vi "Virtual Index of Element in Incremental Array.vi"(9 "Value":dbl, 11 "Incremental Array":dbl[](array[numeric])) -> (0 "Valid Array":bool, 1 "Virtual Index":dbl)   [LabVIEW 2021, in "Arrays.lvlib"]
uses:
  Arrays.lvlib
  bfce6fbf-d7d3-4d45-9a31-a5a003d58b92.vi
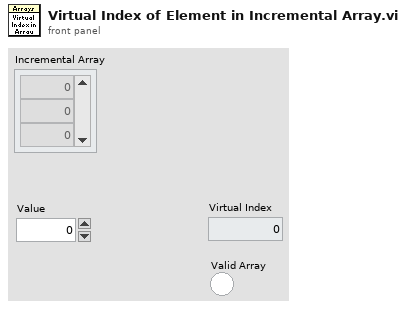
[diagram p1: front panel]
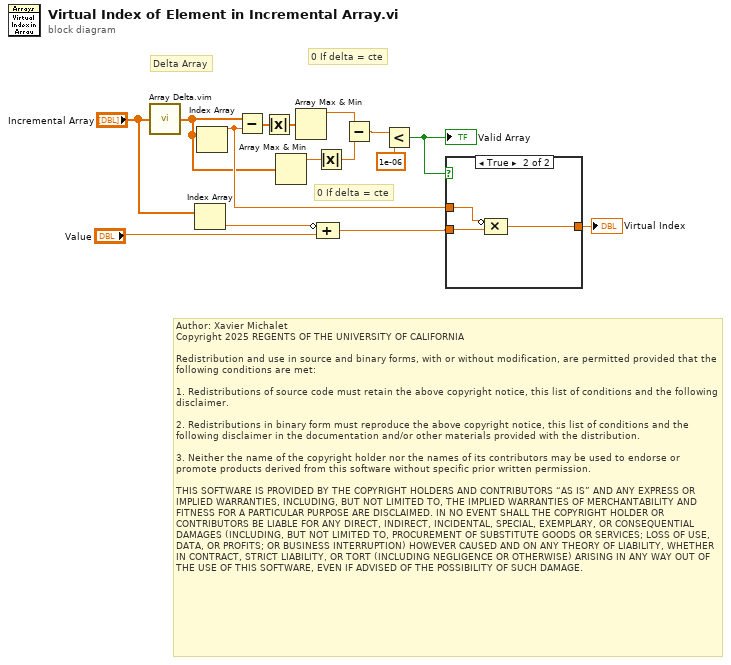
[diagram p0: block diagram]
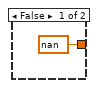
[diagram p2: hidden frame]
diagram:
  # "Author: Xavier Michalet\nCopyright 2025 REGENTS OF THE UNIVERSITY OF CALIFORNIA\n\nRedistribution and use in source and binary forms, with or without modification, are permitted provided that the following conditions are met:\n\n1. Redistributions of source code must retain the above copyright notice, this list of conditions and the following disclaimer.\n\n2. Redistributions in binary form must reproduce the above copyright notice, this list of conditions and the following disclaimer in the documentation and/or other materials provided with the distribution.\n\n3. Neither the name of the copyright holder nor the names of its contributors may be used to endorse or promote products derived from this software without specific prior written permission.\n\nTHIS SOFTWARE IS PROVIDED BY THE COPYRIGHT HOLDERS AND CONTRIBUTORS “AS IS” AND ANY EXPRESS OR IMPLIED WARRANTIES, INCLUDING, BUT NOT LIMITED TO, THE IMPLIED WARRANTIES OF MERCHANTABILITY AND FITNESS FOR A PARTICULAR PURPOSE ARE DISCLAIMED. IN NO EVENT SHALL THE COPYRIGHT HOLDER OR CONTRIBUTORS BE LIABLE FOR ANY DIRECT, INDIRECT, INCIDENTAL, SPECIAL, EXEMPLARY, OR CONSEQUENTIAL DAMAGES (INCLUDING, BUT NOT LIMITED TO, PROCUREMENT OF SUBSTITUTE GOODS OR SERVICES; LOSS OF USE, DATA, OR PROFITS; OR BUSINESS INTERRUPTION) HOWEVER CAUSED AND ON ANY THEORY OF LIABILITY, WHETHER IN CONTRACT, STRICT LIABILITY, OR TORT (INCLUDING NEGLIGENCE OR OTHERWISE) ARISING IN ANY WAY OUT OF THE USE OF THIS SOFTWARE, EVEN IF ADVISED OF THE POSSIBILITY OF SUCH DAMAGE."
  # "0 If delta = cte"
  # "0 If delta = cte"
  # "Delta Array"
  n1 = call "Array Delta.vim"("A"="Incremental Array") -> ("A[i+1]-A[i]"=w8:dbl[])  [unwired: 8 in]
  n2 = Index Array(array="Incremental Array") -> (element=w14:dbl)  [unwired: 1 in]
  n3 = Index Array(array=w8) -> (element=w10:dbl)  [unwired: 1 in]
  n4 = Subtract(x=w8, y=w10) -> (x-y=w9:dbl[])
  n5 = Absolute Value(x=w9) -> (abs(x)=w7:dbl[])
  n6 = Array Max & Min(array=w8) -> (max value=w6:dbl)  [unwired: 3 out]
  n7 = Array Max & Min(array=w7) -> (max value=w2:dbl)  [unwired: 3 out]
  n8 = Absolute Value(x=w6) -> (abs(x)=w1:dbl)
  n9 = Compound Arithmetic op=ADD(invert w14, "Value") -> (w12:dbl)
  n10 = Subtract(x=w2, y=w1) -> (x-y=w5:dbl)
  n11 = Less?(x=w5, y=1e-06) -> (x < y?=w3:bool)
  "Valid Array" <- w3
  n12 = case shown="True" w3 {
    tunnel: w12 -> [_ w19]
    tunnel: w10 -> [_ w18]
    tunnel: [nan w17] -> w11
    frame False {
    }
    frame True {
      n13 = Compound Arithmetic op=MULTIPLY(invert w18, w19) -> (w17:dbl)
    }
  }
  "Virtual Index" <- w11
